vi "Update Filter List.vi"(7 "MCListbox Refnum":refnum<vi>, 8 "error in (no error)":errorcluster, 10 "Filter Array":refnum<class "Base Filter.lvclass">[](array[class])) -> (0 "error out":errorcluster)   [LabVIEW 2016, in "Assert API Components.lvlib" / "Assert Display.lvlib" / "Filter Config Display.lvlib" / "Filter Config Display.lvclass"]
uses:
  Filter Config Display.lvclass
  Assert API Components/Filter Configurations/Base Filter.lvclass
  Assert API Components/Filter Configurations/Base Filter.lvclass/Base Filter.ctl
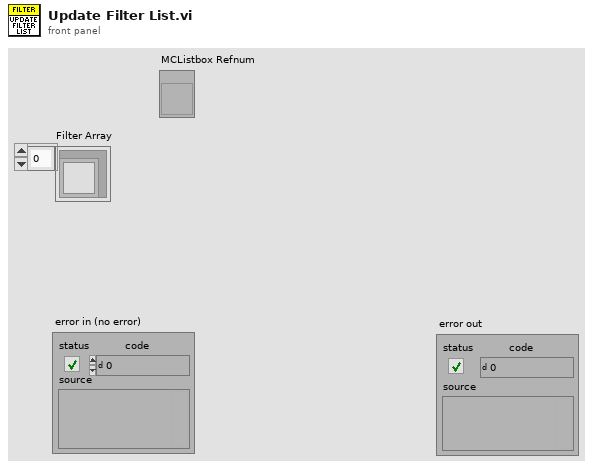
[diagram p1: front panel]
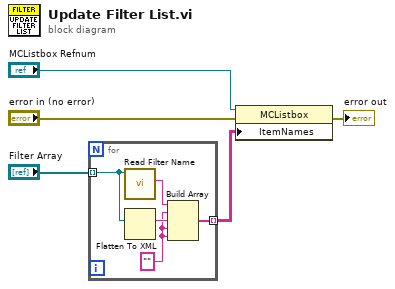
[diagram p0: block diagram]
diagram:
  n1 = for {
    tunnel: "Filter Array" -> [w10] mode=indexing
    tunnel: [w6] -> w1 mode=indexing
    w7 = "" ("element")
    n2 = call "Read Filter Name.vi"("Base Filter in"=w10) -> ("Filter Name"=w9:string)  [unwired: 10 in]
    n3 = Flatten To XML(anything=w10) -> (xml string=w8:string)
    n4 = Build Array(w9, w7, w8, w7, w7) -> (w6:string[])
  }
  n5 = property class="MCListbox"(reference="MCListbox Refnum", error in="error in (no error)", "ItemNames"=w1) -> (error out=→"error out":errorcluster)  [unwired: 1 out]
